vi "MasterDirectory.vi"() -> (0 "Master Directory":path=path "C:/CuspControl")   [LabVIEW 2018]
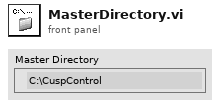
[diagram p1: front panel]
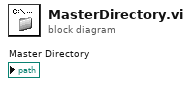
[diagram p0: block diagram]
diagram:
